vi "Export as image by control reference.vi"(8 "error in (no error)":errorcluster, 11 "Ctl Refnum":refnum<vi>) -> (0 "error out":errorcluster, 3 "Image path":path)   [LabVIEW 2016]
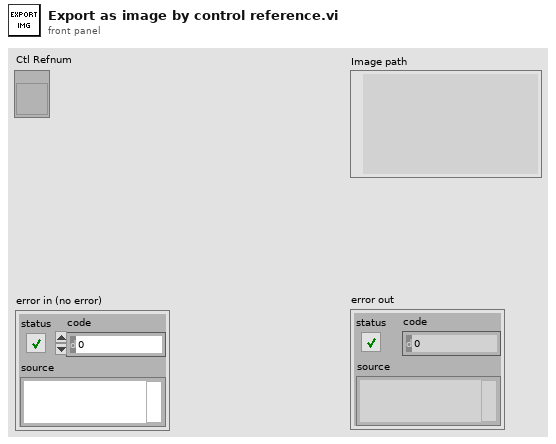
[diagram p1: front panel]
types:
  T1 = typedef "imagedata.ctl" = cluster{"image type":i32, "image depth":i32, "image":u8[], "mask":u8[], "colors":u32[], "Rectangle":cluster{"left":i16, "top":i16, "right":i16, "bottom":i16}}
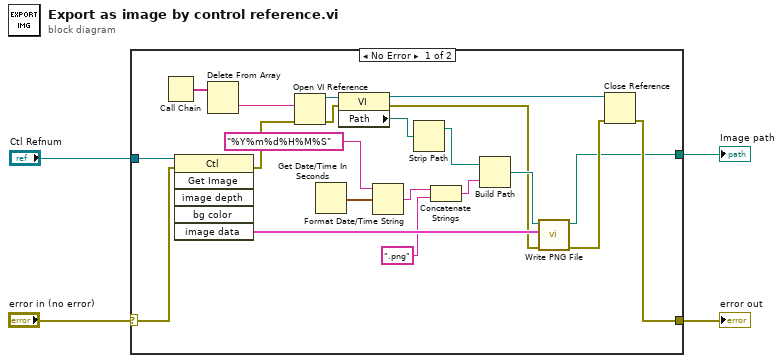
[diagram p0: block diagram]
diagram:
  n1 = case shown="No Error" "error in (no error)" {
    selector: "error in (no error)" -> [w17 w26]
    tunnel: [w15 w26] -> w4
    tunnel: "Ctl Refnum" -> [w25 _]
    tunnel: [w11 _] -> w1
    frame No Error {
      n2 = Call Chain() -> (call chain=w24:string[])
      n3 = invoke class="Ctl" method="Get Image"(reference=w25, error in=w17) -> (error out=w14:errorcluster, "image data"=w22:T1)  [unwired: 4 in, 4 out]
      n4 = Delete From Array(array=w24) -> (deleted portion=w23:string)  [unwired: 2 in, 1 out]
      n5 = Open VI Reference(vi path=w23, error in (no error)=w14) -> (vi reference=w21:refnum<vi>, error out=w13:errorcluster)  [unwired: 4 in]
      n6 = Get Date/Time In Seconds() -> (seconds since 1Jan1904=w20:timestamp)
      n7 = property class="VI"(reference=w21, error in=w13) -> (reference out=w18:refnum<vi>, error out=w12:errorcluster, "Path"=w10:path)
      n8 = Format Date/Time String(time format string (%c)="%Y%m%d%H%M%S", seconds (now)=w20) -> (date/time string=w7:string)  [unwired: 1 in]
      n9 = Strip Path(path=w10) -> (stripped path=w9:path)  [unwired: 1 out]
      n10 = Concatenate Strings(w7, ".png" ("string")) -> (w6:string)
      n11 = Build Path(base path=w9, name or relative path=w6) -> (appended path=w19:path)
      n12 = call <vilib>:"Write PNG File.vi"("error in (no error)"=w12, "image data"=w22, "path to PNG file"=w19) -> ("error out"=w16:errorcluster, "path"=w11:path)  [unwired: 7 in]
      n13 = Close Reference(reference=w18, error in (no error)=w16) -> (error out=w15:errorcluster)
    }
    frame Error {
    }
  }
  "error out" <- w4
  "Image path" <- w1
